vi "AI.vi"(10 "DAQ模拟采集通道参数设置":T1={"数据采集通道设置"={"physical channels"="", "maximum value"=5.0, "minimum value"=-5.0, "input terminal configuration"=-1}, "采样设置"={"rate"=1000.0, "sample mode"=10178, "samples per channel"=1000}, "ConvLateErrorsToWarnings"=FALSE} {"采样设置"."sample mode" items=["Finite Samples"=10178, "Continuous Samples"=10123, "Hardware Timed Single Point"=12522]; "采样设置"."rate" format="%0.2f"; "数据采集通道设置"."input terminal configuration" items=["Default"=-1, "RSE"=10083, "NRSE"=10078, "Differential"=10106, "Pseudodifferential"=12529]; "数据采集通道设置"."minimum value" format="%0.2f"; "数据采集通道设置"."maximum value" format="%0.2f"}) -> (0 "error out":errorcluster, 3 "task out":refnum<k21>)   [LabVIEW 2018]
uses:
  <vilib>/DAQmx/create/channels.llb/DAQmx Create Channel (AI-Voltage-Basic).vi
  <vilib>/DAQmx/configure/timing.llb/DAQmx Timing (Sample Clock).vi
  <resource>/objmgr/daqmx.rc
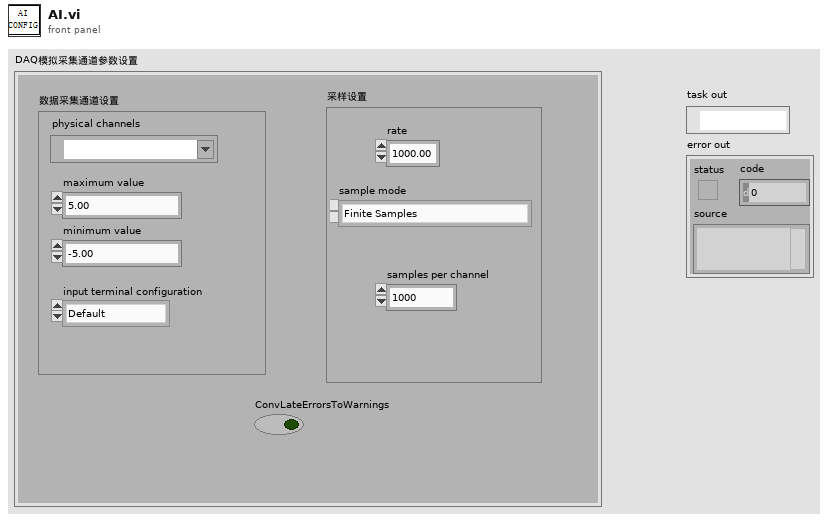
[diagram p1: front panel]
types:
  T1 = cluster{"数据采集通道设置":cluster{"physical channels":tag, "maximum value":dbl, "minimum value":dbl, "input terminal configuration":i32}, "采样设置":cluster{"rate":dbl, "sample mode":i32, "samples per channel":i32}, "ConvLateErrorsToWarnings":bool}
  T2 = cluster{"rate":dbl, "sample mode":i32, "samples per channel":i32}
  T3 = cluster{"physical channels":tag, "maximum value":dbl, "minimum value":dbl, "input terminal configuration":i32}
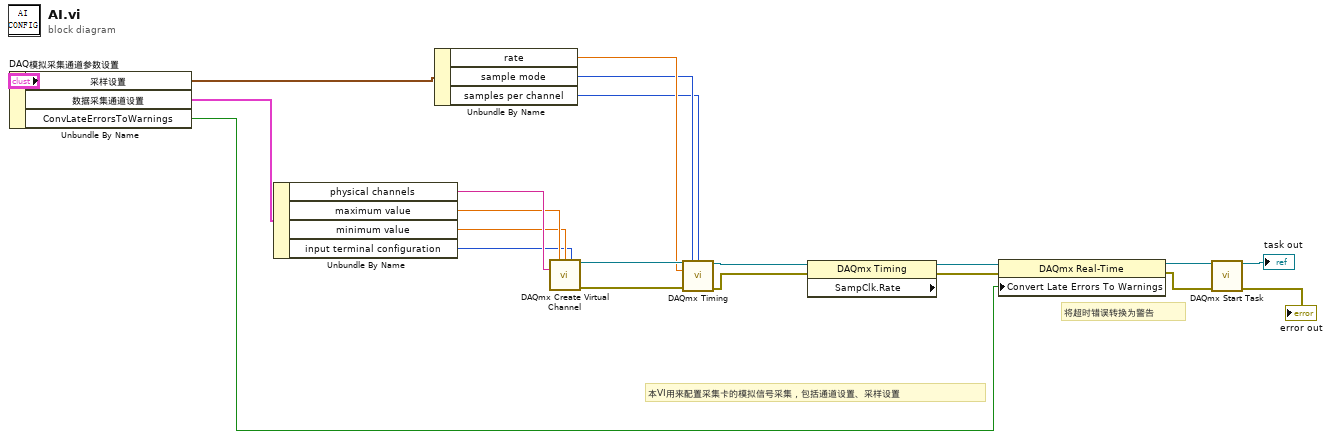
[diagram p0: block diagram]
diagram:
  # "将超时错误转换为警告"
  # "本VI用来配置采集卡的模拟信号采集，包括通道设置、采样设置"
  n1 = Unbundle By Name("DAQ模拟采集通道参数设置") -> ("采样设置"=w2:T2, "数据采集通道设置"=w3:T3, "ConvLateErrorsToWarnings"=w1:bool)
  n2 = Unbundle By Name(w3) -> ("physical channels"=w11:tag, "maximum value"=w10:dbl, "minimum value"=w9:dbl, "input terminal configuration"=w8:i32)
  n3 = Unbundle By Name(w2) -> ("rate"=w7:dbl, "sample mode"=w6:i32, "samples per channel"=w5:i32)
  n4 = call-poly <vilib>:"DAQmx Create Virtual Channel.vi"("maximum value"=w10, "minimum value"=w9, "input terminal configuration"=w8, "physical channels"=w11) -> ("task out"=w19:refnum<k21>, "error out"=w18:errorcluster)  [unwired: 10 in]
  n5 = call-poly <vilib>:"DAQmx Timing.vi"("task/channels in"=w19, "sample mode"=w6, "samples per channel"=w5, "rate"=w7, "error in"=w18) -> ("task out"=w17:refnum<k21>, "error out"=w16:errorcluster)  [unwired: 9 in]
  n6 = property class="DAQmx Timing" props=["SampClk.Rate"](reference=w17, error in=w16) -> (reference out=w21:refnum<k21>, error out=w20:errorcluster)  [unwired: 1 out]
  n7 = property class="DAQmx Real-Time"(reference=w21, error in=w20, "Convert Late Errors To Warnings"=w1) -> (reference out=w15:refnum<k21>, error out=w14:errorcluster)
  n8 = call <vilib>:"DAQmx Start Task.vi"("task/channels in"=w15, "error in"=w14) -> ("task out"=→"task out":refnum<k21>, "error out"=→"error out":errorcluster)  [unwired: 12 in]
